vi "Command-CreateWindow.vi"(8 "error in (no error)":errorcluster, 10 "Data":T1, 11 "Engine in":refnum<class "Engine.lvclass">) -> (3 "Engine out":refnum<class "Engine.lvclass">)   [LabVIEW 2020, in "GLF.lvlib" / "Engine.lvclass"]
uses:
  Engine.lvclass
  Window/Window.lvclass
  Engine.lvclass/Engine.ctl
  Command-CreateWindow--cluster.ctl
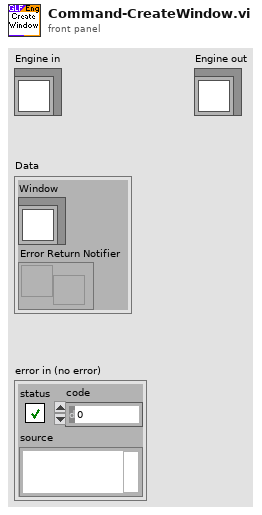
[diagram p1: front panel]
types:
  T1 = typedef "GLF.lvlib/Engine.lvclass/Command-CreateWindow--cluster.ctl" = cluster{"Window":refnum<class "Window.lvclass">, "Error Return Notifier":refnum<notifier>}
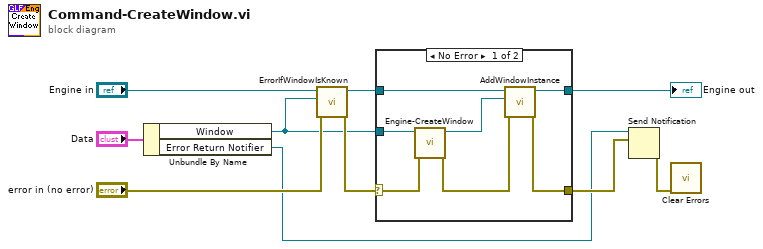
[diagram p0: block diagram]
diagram:
  n1 = Unbundle By Name("Data") -> ("Window"=w2:refnum<class "Window.lvclass">, "Error Return Notifier"=w1:refnum<notifier>)
  n2 = call "ErrorIfWindowIsKnown.vi"("error in (no error)"="error in (no error)", "Window"=w2, "GLF Engine in"="Engine in") -> ("error out"=w9:errorcluster, "GLF Engine out"=w3:refnum<class "Engine.lvclass">)  [unwired: 7 in]
  n3 = case shown="No Error" w9 {
    selector: w9 -> [w17 w18]
    tunnel: [w16 w19] -> w8
    tunnel: [w14 w18] -> w6
    tunnel: w3 -> [w13 w19]
    tunnel: w2 -> [w12 _]
    frame No Error {
      n4 = call "Engine-CreateWindow.vi"("error in (no error)"=w17, "Window in"=w12) -> ("error out"=w15:errorcluster, "Window out"=w11:refnum<class "Window.lvclass">)  [unwired: 6 in, 2 out]
      n5 = call "AddWindowInstance.vi"("error in (no error)"=w15, "Window Instance"=w11, "Engine in"=w13) -> ("error out"=w14:errorcluster, "Engine out"=w16:refnum<class "Engine.lvclass">)  [unwired: 7 in]
    }
    frame Error {
    }
  }
  "Engine out" <- w8
  n6 = Send Notification(notification=w6, notifier=w1) -> (error out=w5:errorcluster)  [unwired: 1 in, 1 out]
  n7 = call <vilib>:"Clear Errors.vi"("error in (no error)"=w5) -> ()  [unwired: 5 in, 2 out]
